vi "array.vi"(11 "input":dbl[](array[numeric])) -> (3 "output":dbl[](array[numeric]))   [LabVIEW 2020]
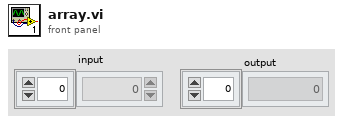
[diagram p1: front panel]
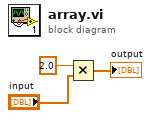
[diagram p0: block diagram]
diagram:
  n1 = Multiply(x=2.0, y="input") -> (x*y=→"output":dbl[])
